vi "Main_23a.vi"() -> ()   [LabVIEW 2023]
uses:
  RB ENUM_Type.ctl
panel:
  out "Array":T1[][](array[typedef])
  out "Position":T1
  out "Answer":u32
  in  "Puzzle":string="#.###########################################################################################################################################\n#...#.....#.....................#...#.........###...###...###...#...#.......#...###.....#...#.......###.........#...........#.............###\n###.#.###.#.###################.#.#.#.#######.###.#.###.#.###.#.#.#.#.#####.#.#.###.###.#.#.#.#####.###.#######.#.#########.#.###########.###\n#...#...#...###...#.............#.#.#.......#.....#...#.#.#...#...#.#.....#.#.#...#...#...#...#...#.#...#.......#.........#.#.#.........#...#\n#.#####.#######.#.#.#############.#.#######.#########.#.#.#.#######.#####.#.#.###.###.#########.#.#.#.###.###############.#.#.#.#######.###.#\n#.......###...#.#.#...............#...#.....#.........#.#...#.......#.....#...#...###.....#...#.#...#...#.#...###...###...#.#.#.#...###.....#\n###########.#.#.#.###################.#.#####.#########.#####.#######.#########.#########.#.#.#.#######.#.#.#.###.#.###.###.#.#.#.#.#########\n#.........#.#...#.....................#.....#.###.....#.....#...#...#.......#...#...#####...#.#.#...###.#.#.#.....#...#.#...#.#...#.........#\n#.#######.#.###############################.#.###.###.#####.###.#.#.#######.#.###.#.#########.#.#.#.###.#.#.#########.#.#.###.#############.#\n#.......#...#.....###.....#...###.....###...#...#.#...#...#.#...#.#.....#...#...#.#.###...#...#...#.#...#.#.#.....#...#.#...#.#.............#\n#######.#####.###.###.###.#.#.###.###.###.#####.#.#.###.#.#.#.###.#####.#.#####.#.#.###.#.#.#######.#.###.#.#.###.#.###.###.#.#.#############\n#.....#.....#.#...#...#...#.#...#...#...#.#...#...#...#.#.#.#...#.....#.#.#.....#.#.###.#.#...#.....#...#.#...#...#.###.#...#.#.......#...###\n#.###.#####.#.#.###.###.###.###.###.###.#.#.#.#######.#.#.#.###.#####.#.#.#.#####.#.###.#.###.#.#######.#.#####.###.###.#.###.#######.#.#.###\n#...#.......#.#...#...#...#.#...###...#.#.#.#.........#.#.#.#...#...#.#.#.#.###...#.#...#.....#.###...#.#.#...#...#...#.#...#.#.......#.#.###\n###.#########.###.###.###.#.#.#######.#.#.#.###########.#.#.#.###.#.#.#.#.#.###.###.#.#########.###.#.#.#.#.#.###.###.#.###.#.#.#######.#.###\n###.....#...#.#...###...#.#.#.#.>.>...#.#.#...#.......#.#.#.#.###.#.#.#.#.#.###.#...#.........#...#.#.#.#...#.>.>.#...#...#.#.#.....#...#...#\n#######.#.#.#.#.#######.#.#.#.#.#v#####.#.###.#.#####.#.#.#.#.###.#.#.#.#.#.###.#.###########.###.#.#.#.#######v###.#####.#.#.#####.#.#####.#\n#...###...#...#.#.....#.#.#.#.#.#.#...#...#...#...#...#.#.#.#.###.#.#.#.#.#.###.#.#...###...#...#.#.#.#.#.....#.#...#...#.#.#.#.....#...#...#\n#.#.###########v#.###.#.#.#.#.#.#.#.#.#####.#####.#.###.#.#.#.###.#.#.#.#.#.###.#.#.#.###.#.###.#.#.#.#.#.###.#.#.###.#.#.#.#.#.#######.#.###\n#.#.....#...###.>.###.#.#.#.#.#.#.#.#...###.....#.#.#...#.#.#.>.>.#.#.#.#.#...#.#.#.#.>.>.#...#.#.#.#...#...#.#.#...#.#.#.#.#.#...###...#...#\n#.#####.#.#.###v#####.#.#.#.#.#.#.#.###.#######.#.#.#.###.#.###v###.#.#.#.###.#.#.#.###v#####.#.#.#.#######.#.#.###.#.#.#.#.#.###.###.#####.#\n#.#...#...#.#...###...#.#.#.#.#.#.#.#...#.....#.#.#.#...#.#...#...#...#.#.###.#.#.#.#...#...#...#...###.....#.#...#.#.#.#.#.#.###...#.#.....#\n#.#.#.#####.#.#####.###.#.#.#.#.#.#.#.###.###.#.#.#.###.#.###.###.#####.#.###.#.#.#.#.###.#.###########.#####.###.#.#.#.#.#.#.#####.#.#.#####\n#...#.....#.#.....#.#...#.#.#.#.#.#.#.....#...#...#...#.#.#...###...#...#...#...#...#...#.#.###...#...#.....#...#.#.#.#.#.#...###...#.#.....#\n#########.#.#####.#.#.###.#.#.#.#.#.#######.#########.#.#.#.#######.#.#####.###########.#.#.###.#.#.#.#####.###.#.#.#.#.#.#######.###.#####.#\n###...###.#.#...#.#.#.#...#.#.#.#...###...#.....#.....#.#.#.#.......#.......#.....#.....#.#.#...#...#...#...###.#.#.#.#...###...#...#.#.....#\n###.#.###.#.#.#.#.#.#.#.###.#.#.#######.#.#####.#.#####.#.#.#.###############.###.#.#####.#.#.#########.#.#####.#.#.#.#######.#.###.#.#.#####\n#...#.#...#...#...#...#.#...#...#.......#.......#.......#...#.....#.......###...#.#.......#.#.........#...#...#.#.#.#.....#...#.....#.#.#...#\n#.###.#.###############.#.#######.###############################.#.#####.#####.#.#########.#########.#####.#.#.#.#.#####.#.#########.#.#.#.#\n#...#.#...............#...#...###.....#.......#.....#.....#.....#...#.....#.....#.........#.#...#...#.#...#.#.#...#.#...#.#...........#...#.#\n###.#.###############.#####.#.#######.#.#####.#.###.#.###.#.###.#####.#####.#############.#.#.#.#.#.#v#.#.#.#.#####.#.#.#.#################.#\n#...#...#...#.....#...#...#.#.###...#...#.....#...#.#.#...#...#.#.....#####...........###.#.#.#...#.>.>.#...#...###...#...###...#.........#.#\n#.#####.#.#.#.###.#.###.#.#.#.###.#.#####.#######.#.#.#.#####.#.#v###################.###.#.#.#######v#########.#############.#.#.#######.#.#\n#.#...#...#.#.###...#...#...#...#.#.#...#.......#.#...#...#...#.>.>.....#.......#...#...#.#.#.......#.....#.....#...#...#.....#.#.......#.#.#\n#.#.#.#####.#.#######.#########.#.#.#.#.#######.#.#######.#.#####v#####.#.#####.#.#.###.#.#.#######.#####.#.#####.#.#.#.#.#####.#######.#.#.#\n#.#.#.#...#...#...###.......#...#.#.#.#.###.....#.......#.#...#...#.....#.....#...#.....#...#...###...#...#...###.#...#.#.....#.........#.#.#\n#.#.#v#.#.#####.#.#########.#.###.#.#.#.###.###########.#.###.#.###.#########.###############.#.#####.#.#####.###.#####.#####.###########.#.#\n#.#.#.>.#.###...#...#...#...#...#.#.#.#...#.....#...#...#.....#...#.#.....###.............#...#.......#...###.#...#.....#...#...........#.#.#\n#.#.#v###.###.#####.#.#.#.#####.#.#.#.###.#####.#.#.#.###########.#.#.###.###############.#.#############.###.#.###.#####.#.###########.#.#.#\n#.#.#...#...#.....#.#.#.#.#.....#.#.#...#.#.....#.#...#.......#...#.#.#...#...#...#.......#.............#...#...###.#...#.#.#...#.......#...#\n#.#.###.###.#####.#.#.#.#.#.#####.#.###.#.#v#####.#####.#####.#.###.#.#.###.#.#.#.#.###################.###.#######.#.#.#.#.#.#.#.###########\n#.#.###...#.....#.#.#.#.#.#.#...#.#...#.#.>.>...#.......#.....#...#.#.#.###.#.#.#.#...###...#...#.....#...#...#.....#.#.#.#.#.#.#...#...#...#\n#.#.#####.#####.#.#.#.#.#.#.#.#.#.###.#.###v###.#########.#######.#.#.#.###.#.#.#.###v###.#.#.#.#.###.###.###.#.#####.#.#.#.#.#.###v#.#.#.#.#\n#...#.....#...#...#...#.#.#.#.#.#...#.#.###...#.#...#...#...###...#...#...#.#.#.#...>.>.#.#.#.#.#.###.....#...#.....#.#.#.#.#.#.#.>.#.#...#.#\n#####.#####.#.#########.#.#.#.#.###.#.#.#####.#.#.#.#.#.###.###.#########.#.#.#.#####v#.#.#.#.#.#.#########.#######.#.#.#.#.#.#.#.#v#.#####.#\n#.....#...#.#.#.......#.#.#...#.#...#...#.....#...#...#.#...#...#...#####...#.#.###...#.#.#.#.#.#.#.......#.......#.#.#.#.#...#...#...#...#.#\n#.#####.#.#.#.#.#####.#.#.#####.#.#######.#############.#.###.###.#.#########.#.###.###.#.#.#.#.#.#.#####.#######.#.#.#.#.#############.#.#.#\n#.......#...#...#.....#...#.....#.###...#...........###.#.#...#...#.........#...#...###...#.#.#.#.#.....#.......#.#...#...#.............#...#\n#################.#########.#####.###.#.###########.###.#.#.###.###########.#####.#########.#.#.#.#####.#######.#.#########.#################\n#.............#...#...#...#.#.....#...#...#.........#...#.#...#.#.......#...###...#.......#.#.#.#.#...#.......#...#.......#.................#\n#.###########.#.###.#.#.#.#.#.#####.#####.#.#########.###.###.#.#.#####.#.#####.###.#####.#.#.#.#.#.#.#######.#####.#####.#################.#\n#...........#...###.#.#.#.#...#...#.....#...#...#...#...#...#...#.....#.#.#.....###.#.....#...#.#.#.#.........###...#...#...#...............#\n###########.#######.#.#.#.#####.#.#####.#####.#.#.#.###.###.#########.#.#.#.#######.#.#########.#.#.#############.###.#.###.#.###############\n#...........#.......#...#.#...#.#.#...#.......#...#...#.#...###.......#...#.........#...###...#...#.............#...#.#.....#...........#...#\n#.###########.###########.#.#.#.#.#.#.###############.#.#.#####.#######################.###.#.#################.###.#.#################.#.#.#\n#...#.........#...........#.#.#.#.#.#.#...#.........#.#...#...#.........#.............#...#.#.#...#.........#...###.#.....#...#...###...#.#.#\n###.#.#########.###########.#.#.#.#.#.#.#.#.#######.#.#####.#.#########.#.###########.###.#.#.#.#.#.#######.#.#####.#####.#.#.#.#.###v###.#.#\n###.#.#.....#...#...#.....#.#.#.#.#.#.#.#...#...###...#...#.#.#...#.....#...........#.#...#.#...#.#.....#...#.....#...#...#.#.#.#.#.>.###.#.#\n###.#.#.###.#.###.#v#.###.#.#.#.#.#.#.#.#####.#.#######.#.#.#.#.#.#.###############.#.#.###.#####.#####.#.#######.###.#.###.#.#.#.#.#v###.#.#\n#...#.#...#...#...#.>.#...#.#.#.#.#.#.#.......#.....#...#.#.#...#...#.......#.......#...#...#.....###...#.........#...#.#...#.#.#.#.#.....#.#\n#.###.###.#####.###v###.###.#.#.#.#.#.#############.#.###.#.#########.#####.#.###########.###.#######.#############.###.#.###.#.#.#.#######.#\n#.....###.......#...###...#.#.#.#.#.#.###...........#...#.#...........#.....#...#.....###...#.#.....#.#...#.....#...#...#...#...#...#.....#.#\n#################.#######.#.#.#.#.#.#.###.#############.#.#############.#######.#.###.#####.#.#.###.#.#.#.#.###.#.###.#####.#########.###.#.#\n#.................###.....#.#.#.#.#.#...#...#.........#.#...#...........#...###.#.#...#...#.#.#.#...#...#...#...#...#.#.....#...#.....#...#.#\n#.###################.#####.#.#.#.#.###.###v#.#######.#.###.#.###########.#.###v#.#.###.#.#.#.#.#.###########.#####.#.#.#####.#.#.#####.###.#\n#...................#.......#.#.#.#...#...>.>.#.......#.#...#.......#...#.#.#.>.>.#.###.#.#.#.#.#.###...#...#.###...#.#...#...#.#.....#...#.#\n###################.#########.#.#.###.#####v###.#######.#.#########v#.#.#.#.#.#v###.###.#.#.#.#.#.###.#.#.#.#v###.###.###.#.###.#####.###.#.#\n#...................###.....#.#.#.#...#.....###.#.....#.#.......#.>.>.#.#.#.#.#...#.#...#.#.#...#.....#...#.>.>.#...#.#...#...#.#...#...#.#.#\n#.#####################.###.#.#.#.#.###.#######.#.###.#.#######.#.#v###.#.#.#.###.#.#.###.#.#################v#.###.#.#.#####.#.#.#.###.#.#.#\n#.....................#...#.#...#...###.#.....#.#.###.#.....###...#...#.#.#...###.#...###.#.......#.........#.#.#...#...#...#.#.#.#.#...#.#.#\n#####################.###.#.###########.#.###.#.#.###.#####.#########.#.#.#######.#######.#######.#.#######.#.#.#.#######.#.#.#.#.#.#.###.#.#\n#.....................#...#.#...#.....#...#...#.#.#...#.....#...#...#.#.#.#.......###...#.........#.......#.#.#...#.....#.#...#.#.#...#...#.#\n#.#####################.###.#.#.#.###.#####.###.#.#.###.#####.#.#.#.#.#.#.#.#########.#.#################.#.#.#####.###.#.#####.#.#####.###.#\n#.........#...#...#...#...#.#.#.#...#.#...#.###.#.#.....#.....#.#.#...#.#.#...........#.........#.......#.#...#...#.#...#.....#...#...#.....#\n#########.#.#.#.#v#.#.###.#.#.#.###.#.#.#.#v###.#.#######.#####.#.#####.#.#####################.#.#####.#.#####.#.#.#.#######v#####.#.#######\n#.......#...#...#.>.#...#.#.#.#.#...#.#.#.>.>.#...#...###...###.#.....#...#####.................#.....#...#...#.#.#.#.....#.>.#...#.#.#...###\n#.#####.#########v#####.#.#.#.#.#.###.#.###v#.#####.#.#####.###.#####.#########.#####################.#####.#.#.#.#.#####.#.#v#.#.#.#.#.#.###\n#.....#.###...#...#####.#.#...#.#...#...###.#...#...#.#...#...#.......###...#...#...###...#...###...#.###...#.#.#.#...#...#.#...#...#...#...#\n#####.#.###.#.#.#######.#.#####.###.#######.###.#.###.#.#.###.###########.#.#.###.#.###.#.#.#.###.#.#v###.###.#.#.###.#.###.###############.#\n#.....#.....#.#.......#.#.#.....#...#...#...#...#.#...#.#.#...###...#...#.#.#.....#.#...#...#.#...#.>.>.#.###.#.#...#.#.....#.......#.......#\n#.###########.#######.#.#.#.#####.###.#.#.###.###.#.###.#.#.#####.#.#.#.#.#.#######v#.#######.#.#####v#.#.###.#.###.#.#######.#####.#.#######\n#.......#...#.#.......#...#...#...#...#.#...#.#...#...#.#.#.#...#.#.#.#.#.#.#...#.>.>.#.....#.#...###.#...#...#...#.#.#.......#...#.#.....###\n#######.#.#.#.#.#############.#.###.###.###.#.#.#####.#.#.#.#.#.#.#.#.#.#.#.#.#.#.#v###.###.#.###.###.#####.#####.#.#.#.#######.#.#.#####.###\n#...###...#.#.#.............#...#...#...#...#.#...#...#.#.#.#.#.#.#.#.#...#.#.#.#.#.###...#.#...#.#...#...#.......#...#.........#.#.#...#...#\n#.#.#######.#.#############.#####.###.###.###.###.#.###.#.#v#.#.#.#.#.#####.#.#.#.#.#####.#.###.#.#.###.#.#######################.#.#.#.###.#\n#.#.........#...............###...###...#...#.....#.....#.>.>.#...#.#.....#...#...#.......#...#...#.....#.....#...................#...#.....#\n#.#############################.#######.###.###############v#######.#####.###################.###############.#.#############################\n#.........#.............#.......###...#.#...###...#...#...#.###...#...#...#.................#.#...............#.........#...............#...#\n#########.#.###########.#.#########.#.#.#.#####.#.#.#.#.#.#.###.#.###.#.###.###############.#.#.#######################.#.#############.#.#.#\n#.......#...#...........#...........#.#.#...#...#...#.#.#.#.....#...#...###...............#.#.#.#.............###.......#.#.............#.#.#\n#.#####.#####.#######################.#.###.#.#######.#.#.#########.#####################.#.#.#.#.###########.###.#######.#.#############.#.#\n#.....#.....#...........#.............#.....#.......#.#.#.#...#.....#...#.................#...#...###...#...#...#.....#...#...........#...#.#\n#####.#####.###########.#.#########################.#.#.#.#.#.#.#####.#.#.###########################.#.#.#.###.#####.#.#############.#.###.#\n#...#.....#.#...#...#...#.............#...###.......#...#.#.#.#...#...#.#.....#.....#.....#...#.......#...#.#...#.....#.#...#.........#.#...#\n#.#.#####.#.#.#.#.#.#.###############.#.#.###.###########.#.#.###.#.###.#####.#.###.#.###.#.#.#.###########.#.###.#####.#.#.#.#########.#.###\n#.#.......#...#...#...#.......#.......#.#...#...........#.#.#.#...#.#...#...#...###...#...#.#.#...........#...###...#...#.#...#.........#...#\n#.#####################.#####.#.#######.###.###########.#.#.#.#.###.#.###.#.###########.###.#.###########.#########.#.###.#####.###########.#\n#...#...#...#.....#...#.....#.#.......#.#...#...###.....#...#...#...#...#.#...#.......#.#...#.###...#.....#.....###...#...#.....#...........#\n###.#.#.#.#.#.###.#.#.#####.#.#######.#.#.###.#.###.#############.#####.#.###.#.#####.#.#.###.###.#.#.#####.###.#######.###.#####.###########\n###.#.#.#.#...###...#.#.....#.#.......#.#...#.#.#...#...........#...#...#.#...#.....#...#.#...#...#...#####...#...#...#.....#...#...........#\n###.#.#.#.###########.#.#####.#v#######.###.#.#.#.###.#########.###.#.###.#.#######.#####.#.###.#############.###.#.#.#######.#.###########.#\n###.#.#.#.#...........#.....#.>.>.......#...#.#.#.....#.........###.#...#.#.#...###...###.#.###...........#...#...#.#.#.......#.#.....#...#.#\n###.#.#.#.#.###############.###v#########.###.#.#######.###########.###.#.#.#.#.#####.###.#.#############.#.###.###.#.#.#######.#.###.#.#.#.#\n###...#...#.......#...#####.#...#.........#...#...#...#...#.......#...#...#.#.#.......#...#.#...#.........#...#...#.#.#.......#...###...#...#\n#################.#.#.#####.#.###.#########.#####.#.#.###.#.#####.###.#####.#.#########.###.#.#.#.###########.###.#.#.#######.###############\n###...#...###...#...#.###...#...#.#####...#.....#.#.#.#...#.#.....#...#.....#.........#...#.#.#.#.....###...#...#.#.#.###.....#.......#.....#\n###.#.#.#.###.#.#####.###.#####.#.#####.#.#####.#.#.#.#v###.#.#####.###.#############.###.#.#.#.#####v###.#.###.#.#.#.###.#####.#####.#.###.#\n#...#...#...#.#.#.....#...###...#...#...#.#...#.#.#.#.>.>...#...###...#.......#.......#...#.#.#.#...>.>.#.#.#...#.#.#...#.......#.....#...#.#\n#.#########.#.#.#.#####.#####.#####.#.###.#.#.#.#.#.###v#######.#####.#######.#.#######.###.#.#.#.###v#.#.#.#.###.#.###.#########.#######.#.#\n#.........#.#.#.#...#...#...#.#...#...###.#.#...#.#.###.....#...#...#.#.......#.....#...###...#...###.#.#.#.#...#.#.#...#...#...#...#...#.#.#\n#########.#.#.#.###.#.###.#.#.#.#.#######.#.#####.#.#######.#.###.#.#.#.###########v#.###############.#.#.#.###.#.#.#.###.#.#v#.###.#.#.#.#.#\n###...#...#.#.#.#...#.....#.#.#.#.#...###.#.....#.#.#.......#...#.#.#.#...#.......>.>.#...............#...#.....#.#.#...#.#.>.#.....#.#...#.#\n###.#.#.###.#.#.#v#########.#.#.#.#.#.###.#####.#.#.#.#########.#.#.#.###.#.#######v###.#########################.#.###.#.###v#######.#####.#\n#...#.#...#.#.#.#.>.#.....#.#.#.#...#...#.......#...#.........#...#...#...#.#.......###.....#.....#...#.........#.#.#...#.#...###...#.#.....#\n#.###.###.#.#.#.#v#.#.###.#.#.#.#######.#####################.#########.###.#.#############.#.###.#.#.#.#######.#.#.#.###.#.#####.#.#.#.#####\n#...#.....#.#.#.#.#.#...#.#.#.#.#...###.........#.............#.....###.....#.......###...#...#...#.#.#.#.......#...#.....#...#...#...#.....#\n###.#######.#.#.#.#.###.#.#.#.#.#.#.###########.#.#############.###.###############.###.#.#####.###.#.#.#.###################.#.###########.#\n###...#...#.#.#.#.#.....#...#...#.#...#.........#...#...#.......#...#...###...#...#...#.#.....#.....#...#.#...........#.......#.###.........#\n#####.#.#.#.#.#.#.###############.###.#.###########.#.#.#.#######.###.#.###.#.#.#.###.#.#####.###########.#.#########.#.#######.###.#########\n#.....#.#.#...#...###.....#...###...#...###...#####...#...#.......#...#.#...#...#.....#.....#.#...#...###...#.....#...#...#...#...#.........#\n#.#####.#.###########.###.#.#.#####.#######.#.#############.#######.###.#.#################.#.#.#.#.#.#######.###.#.#####.#.#.###.#########.#\n#.......#.#...#...#...#...#.#.....#.......#.#...#...#...###.......#.#...#.#.....###...#...#.#...#.#.#.###...#...#...#...#.#.#.....#.........#\n#########.#.#.#.#.#.###.###.#####.#######.#.###.#.#.#.#.#########.#.#.###.#.###.###.#.#.#.#.#####.#.#.###.#.###v#####.#.#.#.#######.#########\n#.........#.#.#.#.#...#.###.#.....#...#...#.#...#.#.#.#.#...#...#.#.#.###...###...#.#.#.#.#.....#...#...#.#.#.>.>...#.#.#...#...###.......###\n#.#########.#.#.#.###.#.###.#.#####.#.#v###.#.###.#.#.#.#.#.#.#.#v#.#.###########.#.#.#.#.#####.#######.#.#.#.#####.#.#.#####.#.#########v###\n#.........#.#.#.#...#.#...#.#...#...#.>.>...#...#.#.#.#.#.#.#.#.>.>.#.#...#...#...#.#.#.#.#...#.....###.#.#.#...#...#.#...#...#.#.....#.>.###\n#########.#.#.#.###.#.###.#.###.#.#############.#.#.#.#.#.#.#.#######.#.#.#.#.#.###.#.#.#.#.#.#####.###.#.#.###.#.###.###.#.###.#.###.#.#v###\n#.........#.#...#...#...#.#...#.#.#...#.........#.#.#.#...#.#.#.....#...#...#.#.....#.#.#.#.#.#...#...#.#.#.#...#.#...#...#.#...#...#...#...#\n#.#########.#####.#####.#.###.#.#.#.#.#.#########.#.#.#####.#.#.###.#########.#######.#.#.#.#.#.#.###.#.#.#.#.###.#.###.###.#.#####.#######.#\n#.........#.....#.#...#.#.#...#.#...#.#...#.....#.#.#.#.....#.#...#...........#.......#.#...#...#.#...#...#.#...#.#...#...#.#...#...#.......#\n#########.#####.#.#.#.#.#.#.###.#####.###.#.###.#.#.#.#.#####.###.#############.#######.#########.#.#######.###.#.###.###.#.###.#.###.#######\n###.......#...#.#...#...#.#.###.....#.#...#.###.#.#.#.#...#...###.......#.....#.###...#.......#...#.......#.#...#.#...#...#.#...#.###.......#\n###.#######.#.#.#########.#.#######.#.#.###.###.#.#.#.###.#.###########.#.###.#v###.#.#######.#.#########.#.#.###.#.###.###.#.###.#########.#\n#...#...#...#.#...#...#...#.......#...#.....#...#.#...#...#.....###.....#.###.>.>.#.#.#.......#.....#...#.#.#.#...#.#...#...#...#...#.......#\n#.###.#.#.###.###.#.#.#.#########.###########.###.#####.#######.###.#####.#######.#.#.#.###########.#.#.#.#.#.#.###.#.###.#####.###.#.#######\n#.#...#.#.###...#...#.#.#...#...#.###...#.....#...#.....#.....#.#...#...#.#.......#.#.#...#.......#.#.#...#.#.#.#...#.#...#.....#...#.......#\n#.#.###.#.#####.#####.#.#.#.#.#.#.###.#.#.#####.###.#####.###.#.#.###.#.#.#.#######.#.###.#.#####.#.#.#####.#.#.#.###.#.###.#####.#########.#\n#.#.#...#.....#...#...#.#.#.#.#.#.#...#...#...#...#.#...#.#...#.#...#.#.#.#.....#...#...#...#...#.#.#.#.....#.#.#.#...#.#...#...#.#.........#\n#.#.#.#######.###.#.###.#.#.#.#.#.#.#######.#.###.#.#.#.#.#.###.###.#.#.#.#####.#.#####.#####.#.#.#.#.#.#####.#.#.#.###.#.###.#.#.#.#########\n#...#.........###...###...#...#...#.........#.....#...#...#.....###...#...#####...#####.......#...#...#.......#...#.....#.....#...#.........#\n###########################################################################################################################################.#"
  in  "Example":string="#.#####################\n#.......#########...###\n#######.#########.#.###\n###.....#.>.>.###.#.###\n###v#####.#v#.###.#.###\n###.>...#.#.#.....#...#\n###v###.#.#.#########.#\n###...#.#.#.......#...#\n#####.#.#.#######.#.###\n#.....#.#.#.......#...#\n#.#####.#.#.#########v#\n#.#...#...#...###...>.#\n#.#.#v#######v###.###v#\n#...#.>.#...>.>.#.###.#\n#####v#.#.###v#.#.###.#\n#.....#...#...#.#.#...#\n#.#########.###.#.#.###\n#...###...#...#...#.###\n###.###.#.###v#####v###\n#...#...#.#.>.>.#.>.###\n#.###.###.#.###.#.#v###\n#.....###...###...#...#\n#####################.#"
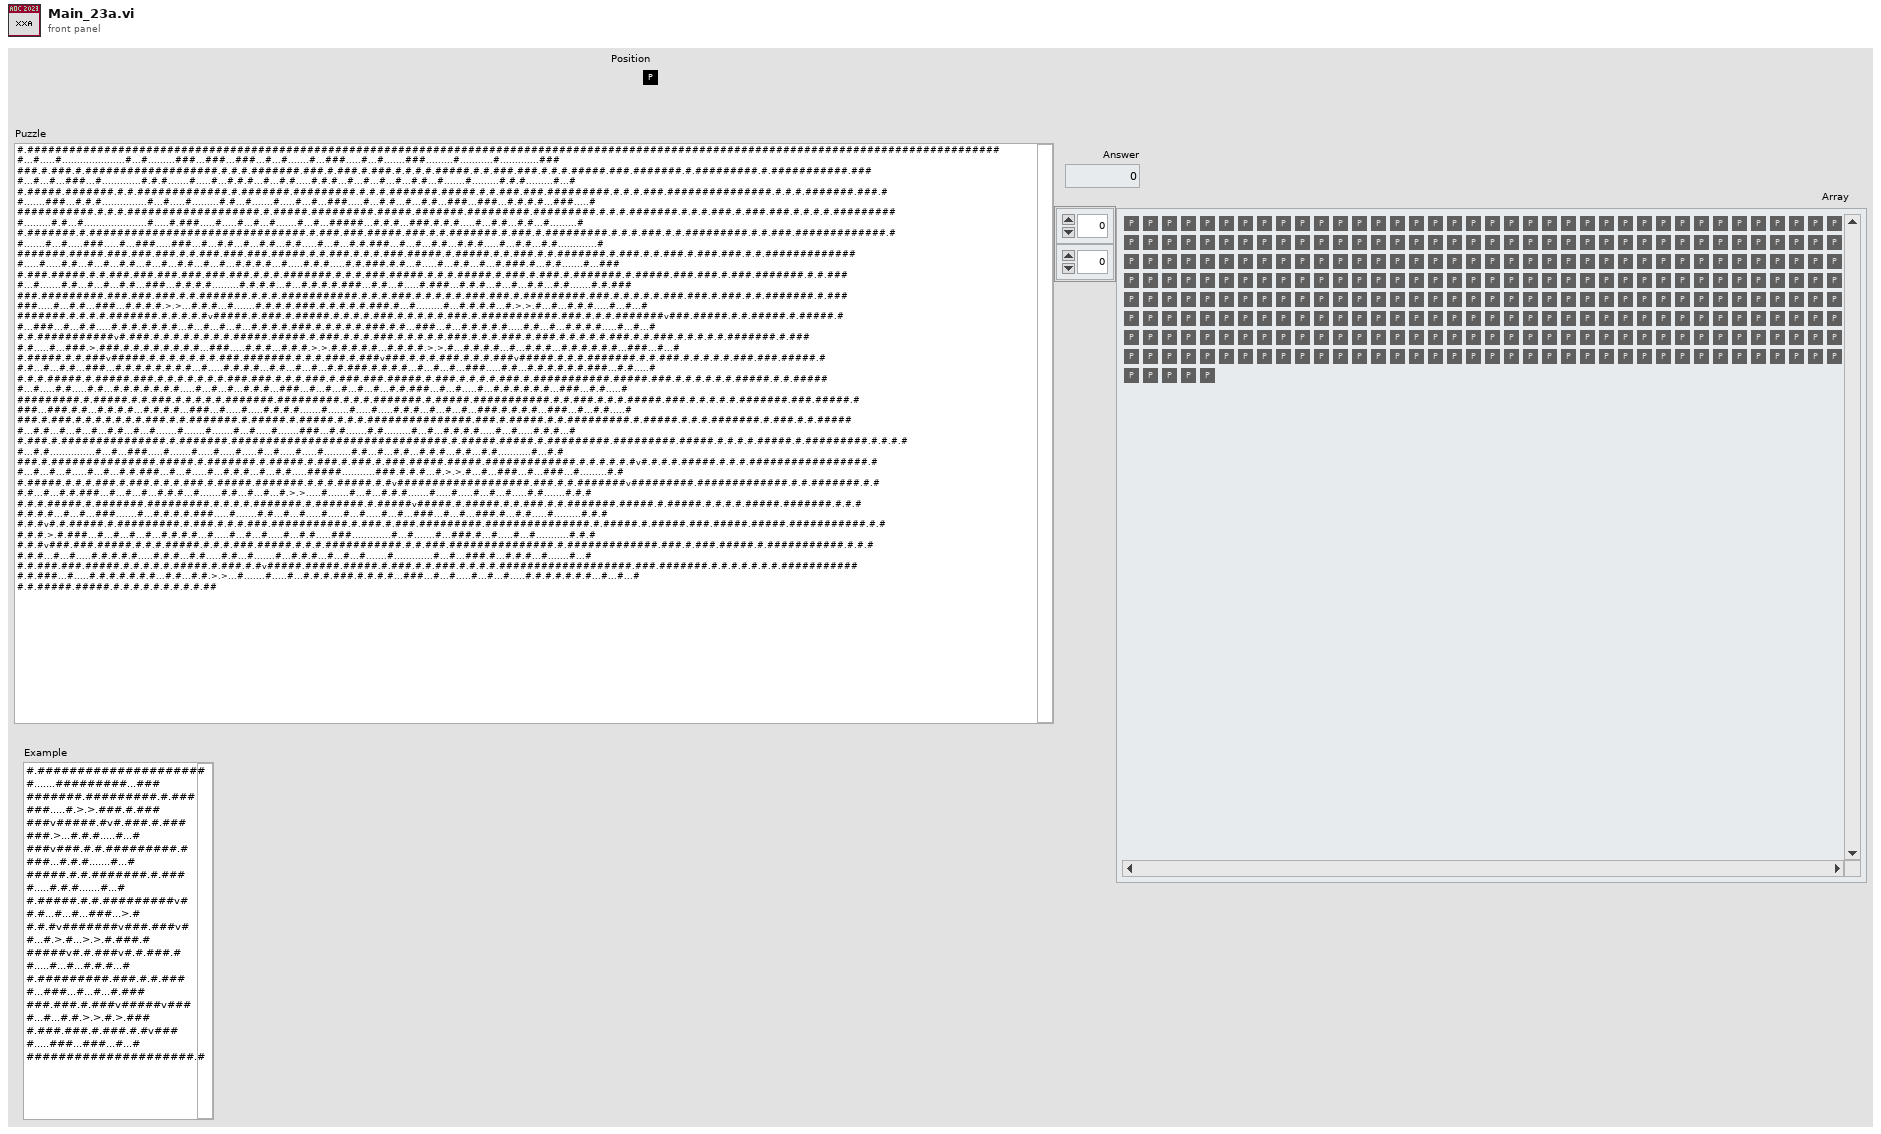
[diagram p1: front panel]
types:
  T1 = typedef "RB ENUM_Type.ctl" = enum32{"Path", "Forest", "UP", "Right", "Down", "Left", "Ocupied"}
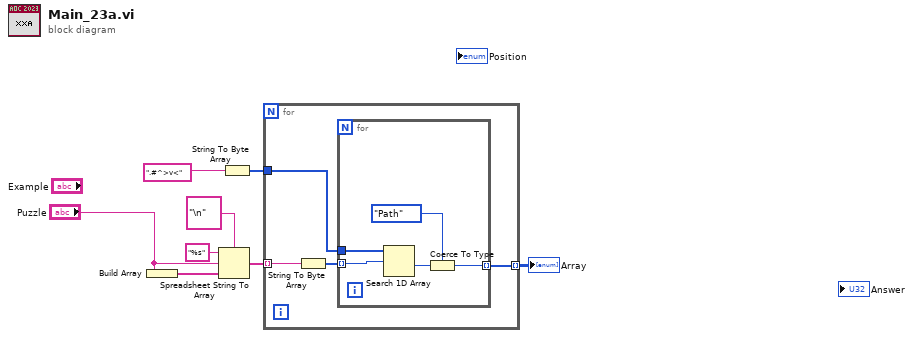
[diagram p0: block diagram]
diagram:
  n1 = Build Array("Puzzle") -> (w8:string[])
  n2 = Spreadsheet String To Array(delimiter (Tab)="\n", format string="%s", spreadsheet string="Puzzle", array type (2D Dbl)=w8) -> (array=w5:string[])
  n3 = String To Byte Array(string=".#^>v<") -> (unsigned byte array=w3:u8[])
  n4 = for {
    tunnel: w5 -> [w12] mode=indexing
    tunnel: w3 -> [w11]
    tunnel: [w9] -> w2 mode=indexing
    n5 = String To Byte Array(string=w12) -> (unsigned byte array=w10:u8[])
    n6 = for {
      tunnel: w11 -> [w17]
      tunnel: w10 -> [w16] mode=indexing
      tunnel: [w13] -> w9 mode=indexing
      n7 = Search 1D Array(1D array=w17, element=w16) -> (index of element=w15:i32)  [unwired: 1 in]
      n8 = Coerce To Type(0:w15, 1:RB_ENUM_Type."Path" ("Position 2")) -> (2:w13:T1)
    }
  }
  "Array" <- w2
